vi "Get as LabVIEW Text.vi"(8 "error in (no error)":errorcluster, 10 "Name Array":string[](array[string]), 11 "JSON Scalar in":refnum<class "JSON Scalar.lvclass">) -> (0 "error out":errorcluster, 1 "Was in quotes":bool, 2 "LabVIEW Text":string, 3 "JSON Scalar out":refnum<class "JSON Scalar.lvclass">)   [LabVIEW 2020, in "Library Commun.lvlib" / "JSON Scalar.lvclass"]
uses:
  JSON Scalar.lvclass
  JSON Scalar.lvclass/JSON Scalar.ctl
  Unescape JSON string.vi
  support/JSON support.lvlib
panel:
  # "Value formated as LabVIEW text:\n-- no quotes on JSON strings\n-- LabVIEW text encoding <ToDo>\n-- no escaped characters <ToDo>"
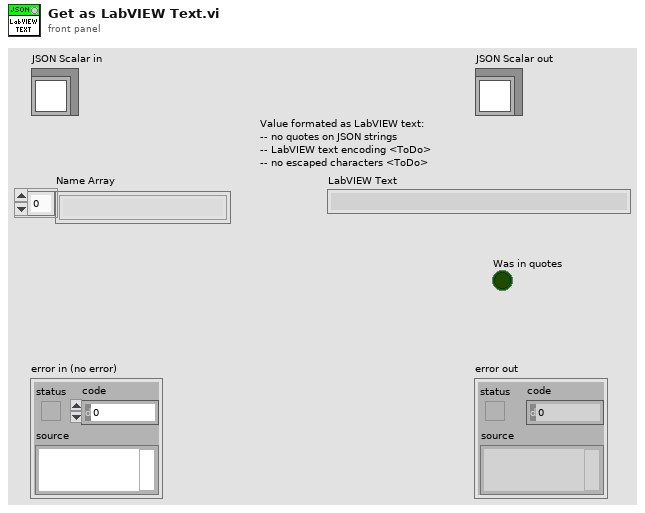
[diagram p1: front panel]
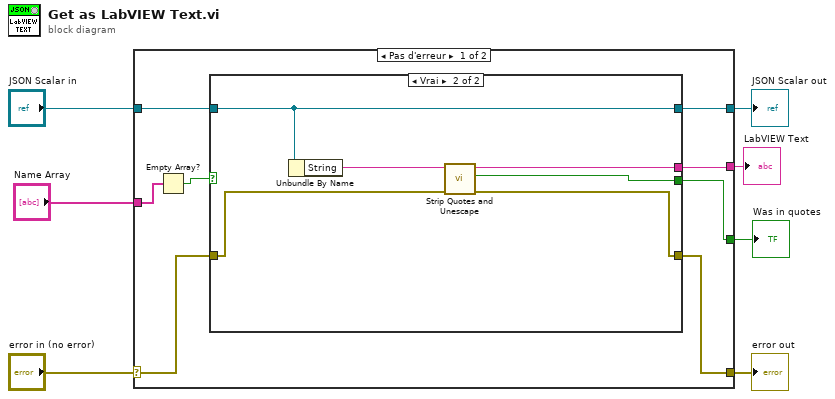
[diagram p0: block diagram]
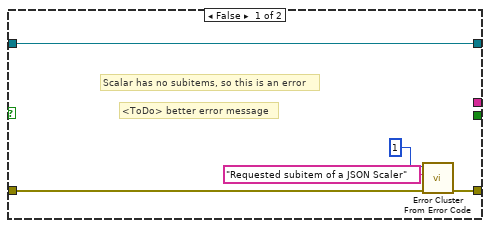
[diagram p2: hidden frame]
diagram:
  n1 = case shown="Pas d'erreur" "error in (no error)" {
    selector: "error in (no error)" -> [w10 w28]
    tunnel: [w9 w28] -> w6
    tunnel: [w11 w27] -> w4
    tunnel: "JSON Scalar in" -> [w12 w27]
    tunnel: [w15 _] -> w3
    tunnel: "Name Array" -> [w14 _]
    tunnel: [w8 _] -> w1
    frame No Error {
      n2 = Empty Array?(array=w14) -> (empty?=w13:bool)
      n3 = case shown="Vrai" w13 {
        tunnel: w12 -> [w20 w24]
        tunnel: [_ w25] -> w15
        tunnel: [w20 w24] -> w11
        tunnel: w10 -> [w16 w23]
        tunnel: [w19 w22] -> w9
        tunnel: [_ w21] -> w8
        frame False {
          # "<ToDo> better error message"
          # "Scalar has no subitems, so this is an error"
          n4 = call <vilib>:"Error Cluster From Error Code.vi"("error in (no error)"=w16, "error message (\"\")"="Requested subitem of a JSON Scaler" ("error message (\"\")"), "error code (0)"=1) -> ("error out"=w19:errorcluster)  [unwired: 6 in]
        }
        frame True {
          n5 = Unbundle By Name(w24) -> ("String"=w26:string)
          n6 = call "Strip Quotes and Unescape.vi"("error in (no error)"=w23, "String"=w26) -> ("error out"=w22:errorcluster, "Had Quotes"=w21:bool, "result string"=w25:string)  [unwired: 7 in]
        }
      }
    }
    frame Error {
    }
  }
  "error out" <- w6
  "JSON Scalar out" <- w4
  "LabVIEW Text" <- w3
  "Was in quotes" <- w1
